vi "Get Column String.vi"(8 "error in (no error)":errorcluster, 11 "PQ Result  in":refnum<class "PQ Result.lvclass">) -> (0 "error out":errorcluster, 2 "String":string, 3 "PQ Result  out":refnum<class "PQ Result.lvclass">)   [LabVIEW 2013, in "PQ Result.lvclass"]
uses:
  PQ Result.lvclass
  PQ Result.lvclass/PQ Result.ctl
  Connection/libpq.dll
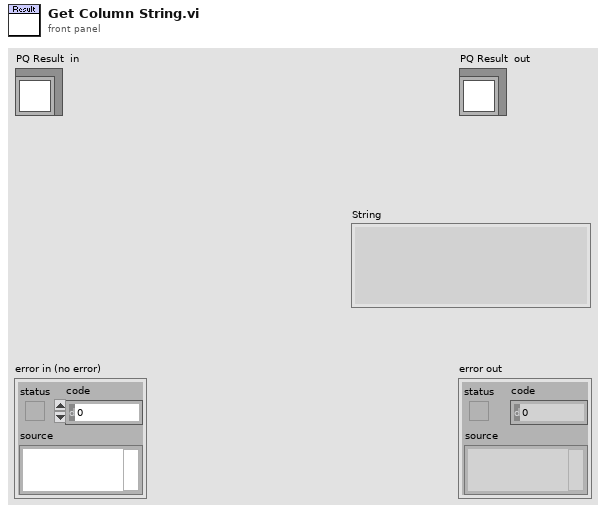
[diagram p1: front panel]
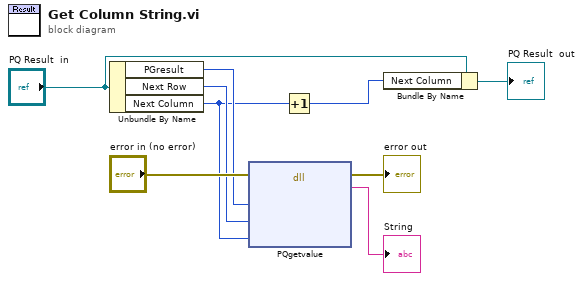
[diagram p0: block diagram]
diagram:
  n1 = Unbundle By Name("PQ Result  in") -> ("PGresult"=w7:u32, "Next Row"=w5:i32, "Next Column"=w3:i32)
  n2 = dll-call lib="C:/Users/patrick/Documents/GitHub/DSC/src/PostgreSQL Library/Connection/libpq.dll" fn="PQgetvalue"(error in="error in (no error)", "PGresult"=w7, "row_number"=w5, "column_number"=w3) -> (error out=→"error out":errorcluster, "PQgetvalue"=→"String":string)  [unwired: 5 in, 1 out]
  n3 = Increment(x=w3) -> (x+1=w2:i32)
  n4 = Bundle By Name(cluster="PQ Result  in", "Next Column"=w2) -> (→"PQ Result  out":refnum<class "PQ Result.lvclass">)
